vi "Periodic Tasks.vi"(8 "error in":errorcluster) -> ()   [LabVIEW 2018]
doc: "This VI runs in parallel to other tasks. It can contain as many user-defined periodic loops as you need. These can carry out PID or other sorts of timed response."
uses:
  State Machines/Intake.ctl
  State Machines/Climber.ctl
  <vilib>/Rock Robotics/WPI/Solenoid/WPI_SolenoidValue.ctl
  <vilib>/Rock Robotics/WPI/ThirdParty/Sensors/navX/_TypeDefs/FRIC_navX_DeviceNumbersTypeDef.ctl
  <vilib>/Rock Robotics/WPI/ThirdParty/Phoenix-LabVIEW/Motor Controller/Controls/CTRE_Phoenix_MotorControl_ControlMode.ctl
  Robot Global Data.vi
  Support Code/Valkyrie1Buttons.vi
  <vilib>/Rock Robotics/WPI/Utilities/WPI_GetSetVariantRefNum.vi
  <vilib>/Rock Robotics/WPI/Solenoid/WPI_SolenoidSetEnum.vi
  <vilib>/Rock Robotics/Network Tables/NT Write Number.vi
  <vilib>/Rock Robotics/Network Tables/NT Write Boolean.vi
panel:
  in  "Value":T1
  out "s? t:f":T1=enum."Forward"
  in  "Score Hatch Angle 2":dbl=12.0
  out "Climber State":T2=enum."cabou"
  in  "Retract back Speed":dbl=-0.4 format="%#_13g"
  in  "Retract Distance":dbl=1400.0 format="%#_13g"
  in  "Retract Speed":dbl=-0.1
  in  "Break speed":dbl=0.2 format="%#_13g"
  in  "Front Limit":dbl=1450.0 format="%#_13g"
  in  "Front Speed":dbl=1.0
  in  "Back Speed":dbl=0.9
  out "Encoder":i32=1460
  in  "Score Angle 2nd":dbl=1.0
  in  "Slow Mode":dbl=0.4
  in  "Cargo Deploy angle 2nd Floor":dbl=1.0
  in  "Cargo 2nd Floor Rocket":dbl=9.5
  in  "Cargo ship height":dbl=9.0
  in  "Cargo 1st Floor Rocket":dbl=5.0 format="%#_13g"
  out "elavador  pos":dbl=-0.00055775
  in  "Height  Hatch 2nd":dbl=9.0
  out "Intake pos":dbl=9.5952787399292
  in  "Turn on point multiplier":dbl=0.6 format="%#_13g"
  in  "Sensitivty":dbl=1.1 format="%#_13g"
  in  "Height Cargo Station":dbl=2.0
  in  "Height Cargo HP":dbl=9.0
  in  "Floor Angle Cargo":dbl=19.0
  in  "Gains":T3={"proportional gain (Kc)"=0.5, "integral time (Ti, min)"=0.1, "derivative time (Td, min)"=0.0} {"derivative time (Td, min)" format="%.3f"; "integral time (Ti, min)" format="%.3f"; "proportional gain (Kc)" format="%.3f"}
  in  "Range":cluster{"output high":dbl, "output low":dbl}={"output high"=1.0, "output low"=-0.4} {"output low" format="%.2f"; "output high" format="%.2f"}
  in  "Disable Range":dbl
  in  "Integral Range":dbl=1.0
  in  "CargoTime":dbl=10.0
  in  "Default height":dbl=3.0 format="%#_13g"
  in  "Cargo Deploy Angle":dbl=10.0
  in  "Tempo de coleta":dbl=7.0 format="%#_13g"
  in  "Sobe":dbl=1.0
  out "Estado Intake":T4
  in  "Desce":dbl=0.3
  in  "Score Hatch Angle":dbl=4.0 format="%#_13g"
  in  "Floor Angle":dbl=20.0
  in  "Hatch intake Speed Floor":dbl=-1.0
  in  "Holding Angle":dbl=4.0
  in  "Hatch intake Speed":dbl=-1.0
  in  "HP Angle 2":dbl=11.0 format="%#_13g"
  in  "HP Angle":dbl=10.0 format="%#_13g"
  in  "Intake Arm PID Constants":T5={"P Gain"=0.15, "I Gain"=1e-05, "D Gain"=5.0, "F Gain"=0.0, "I Zone"=10.0, "Min Output"=-0.2999999999999998, "Max Output"=0.3} {"Max Output" min=-1.0 max=1.0 step=0.01; "Min Output" min=-1.0 max=1.0 step=0.01; "I Zone" step=0.01; "F Gain" step=0.01; "D Gain" step=0.01; "I Gain" step=0.01; "P Gain" min=0.0 step=0.01}
  # "Angles"
  # "Intake Control"
  # "Elevator Control"
  # "Climber"
  # "Drivetrain"
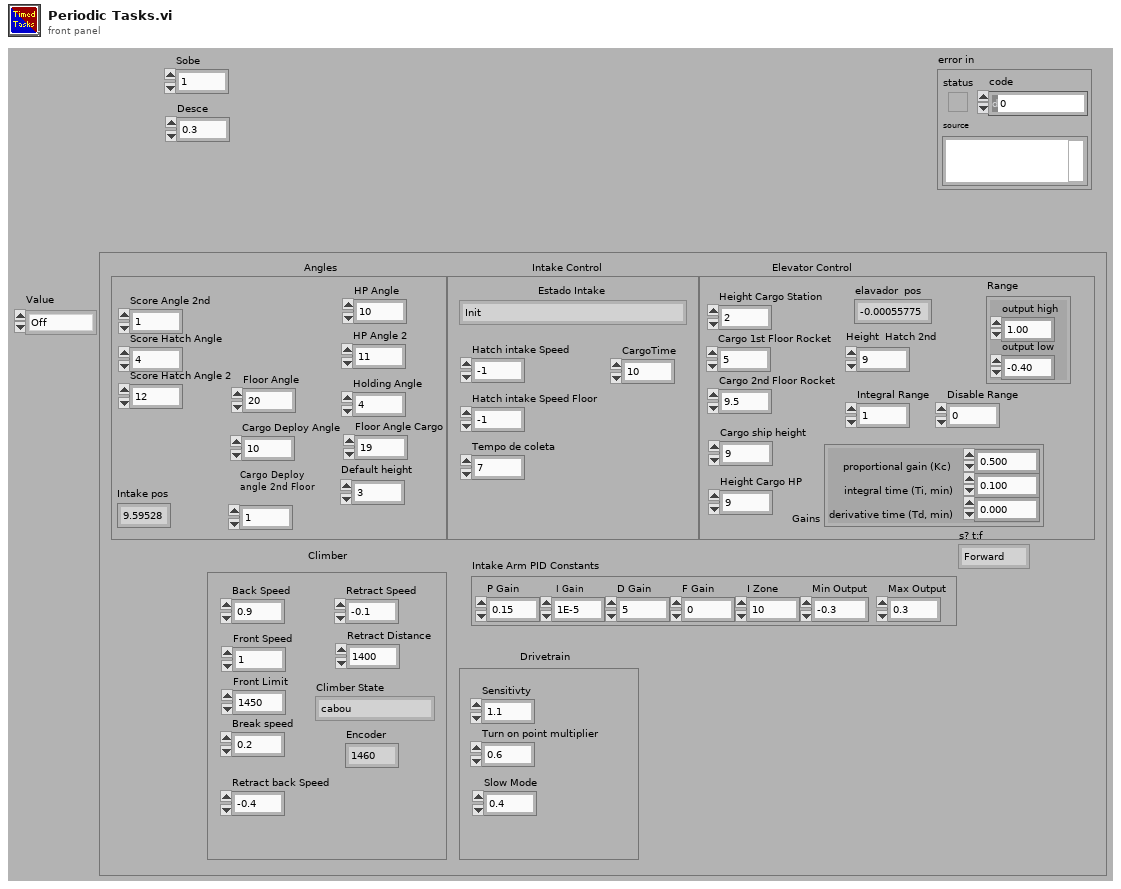
[diagram p1: front panel]
types:
  T1 = typedef "WPI_SolenoidValue.ctl" = enum16{"Off", "On", "Forward", "Reverse"}
  T2 = typedef "Climber.ctl" = enum16{"Engaging Climb", "Wait for Start", "ELEVATE!", "Hold position", "Forward", "Retract varetas", "Charge", "Sobe so um poquinho", "cabou"}
  T3 = cluster{"proportional gain (Kc)":dbl, "integral time (Ti, min)":dbl, "derivative time (Td, min)":dbl}
  T4 = typedef "Intake.ctl" = enum16{"Init", "Preparar Coletar HP", "Coletar Cargo", "Segurando Cargo", "Preparar Score Cargo", "Score Cargo", "Coletar HP", "Coletar Hatch Chão", "Segurando Hatch", "Preparar Score Hatch", "Score Hatch", "Wait"}
  T5 = cluster{"P Gain":dbl, "I Gain":dbl, "D Gain":dbl, "F Gain":dbl, "I Zone":dbl, "Min Output":dbl, "Max Output":dbl}
  T6 = typedef "FRIC_navX_DeviceNumbersTypeDef.ctl" = enum16{"Dev0", "Dev1", "Dev2", "Dev3"}
  T7 = typedef "WPI_MotorControlDeviceRef.ctl" = cluster{"DeviceStatus":errorcluster, "Type":T8, "PWM":cluster{"PWM Channel":T9, "DeadBand":T10}, "CAN":cluster{"Device Number":u8, "SetOutput VI Ref":variant, "GetOutput VI Ref":variant, "Enable VI Ref":variant, "Disable VI Ref":variant, "Data":variant}, "Invert":bool, "DIO PWM":cluster{"PWM \"Enable\" Channel":T9, "DIOChannel":T11, "PWM Rate":dbl}}
  T8 = typedef "WPI_MotorControlType.ctl" = enum16{"PWM", "CAN", "DIO PWM"}
  T9 = typedef "FPGA_DIOPWMChannel.ctl" = enum8{"PWM 0", "PWM 1", "PWM 2", "PWM 3", "PWM 4", "PWM 5", "PWM 6", "PWM 7", "PWM 8", "PWM 9", "PWM MXP 0", "PWM MXP 1", "PWM MXP 2", "PWM MXP 3", "PWM MXP 4", "PWM MXP 5", "PWM MXP 6", "PWM MXP 7", "PWM MXP 8", "PWM MXP 9", "Invalid"}
  T10 = typedef "WPI_PWMDeadband.ctl" = cluster{"Name":string, "maxPositivePwm":i32, "minPositivePwm":i32, "centerPwm":i32, "maxNegativePwm":i32, "minNegativePwm":i32, "angularRange":u16}
  T11 = typedef "FPGA_DIOChannel.ctl" = enum8{"DIO 0", "DIO 1", "DIO 2", "DIO 3", "DIO 4", "DIO 5", "DIO 6", "DIO 7", "DIO 8", "DIO 9", "DIO MXP 0", "DIO MXP 1", "DIO MXP 2", "DIO MXP 3", "DIO MXP 4", "DIO MXP 5", "DIO MXP 6", "DIO MXP 7", "DIO MXP 8", "DIO MXP 9", "DIO MXP 10", "DIO MXP 11", "DIO MXP 12", "DIO MXP 13", "DIO MXP 14", "DIO MXP 15", "SPI Port CS1", "SPI Port CS2", "SPI Port CS3", "SPI Port MISO", "SPI Port MOSI", "Invalid"}
  T12 = typedef "Button Cluster.ctl" = cluster{"Buttons[0]":bool, "Buttons[1]":bool, "Buttons[2]":bool, "Buttons[3]":bool, "Buttons[4]":bool, "Buttons[5]":bool, "Buttons[6]":bool, "Buttons[7]":bool, "Buttons[8]":bool, "Buttons[9]":bool}
  T13 = typedef "WPI_SwitchDevRef.ctl" = cluster{"DevStatus":errorcluster, "DIO Channel":T11, "CntIndex":T14, "Normally Closed":bool}
  T14 = typedef "FPGA_CounterCtrSystemIndex.ctl" = enum8{"Ctr 0", "Ctr 1", "Ctr 2", "Ctr 3", "Ctr 4", "Ctr 5", "Ctr 6", "Ctr 7", "Invalid"}
  T15 = typedef "WPI_SolenoidDevRef.ctl" = cluster{"DevStatus":errorcluster, "Pneumatics Control Module":u8, "Forward Solenoid Channel":T16, "Reverse Solenoid Channel":T16}
  T16 = typedef "WPI_SolenoidChannel.ctl" = enum8{"Solenoid 0", "Solenoid 1", "Solenoid 2", "Solenoid 3", "Solenoid 4", "Solenoid 5", "Solenoid 6", "Solenoid 7", "Invalid"}
  T17 = typedef "WPI_EncoderDevRef.ctl" = cluster{"DevStatus":errorcluster, "EncoderIndex":T18, "CounterIndex":T14, "DistancePerCount":dbl, "Decoding Type":T19}
  T18 = typedef "FPGA_EncoderIdx.ctl" = enum8{"Enc 0", "Enc 1", "Enc 2", "Enc 3", "Enc 4", "Enc 5", "Enc 6", "Enc 7", "Invalid"}
  T19 = typedef "WPI_EncoderType.ctl" = enum16{"1x", "2x", "4x"}
  T20 = typedef "CTRE_Phoenix_MotorControl_ControlMode.ctl" = u16
  T21 = typedef "WPI_CounterDevRef.ctl" = cluster{"DevStatus":errorcluster, "CntIndex":T14}
  T22 = typedef "WPI_RobotDriveDevRef.ctl" = cluster{"DevStatus":errorcluster, "Motors[]":T7[], "Square Inputs":bool, "Max Output":dbl}
  T23 = typedef "Axes Cluster.ctl" = cluster{"Axes[0]":dbl, "Axes[1]":dbl, "Axes[2]":dbl, "Axes[3]":dbl, "Axes[4]":dbl, "Axes[5]":dbl, "Axes[6]":dbl, "Axes[7]":dbl, "Axes[8]":dbl}
  T24 = typedef "D-Pad.ctl" = cluster{"Top":bool, "Bottom":bool, "None":bool, "Right":bool, "Left":bool}
  T25 = typedef "WPI_CompressorDevRef.ctl" = cluster{"DevStatus":errorcluster, "Pneumatics Control Module":u8}
  T26 = typedef "WPI_JoystickDevRef.ctl" = cluster{"Device":T27}
  T27 = typedef "WPI_JoystickDeviceEnum.ctl" = enum16{"USB 0", "USB 1", "USB 2", "USB 3", "USB 4", "USB 5"}
  T28 = cluster{"Rollover":dbl, "Yaw":dbl, "Cont Yaw":dbl}
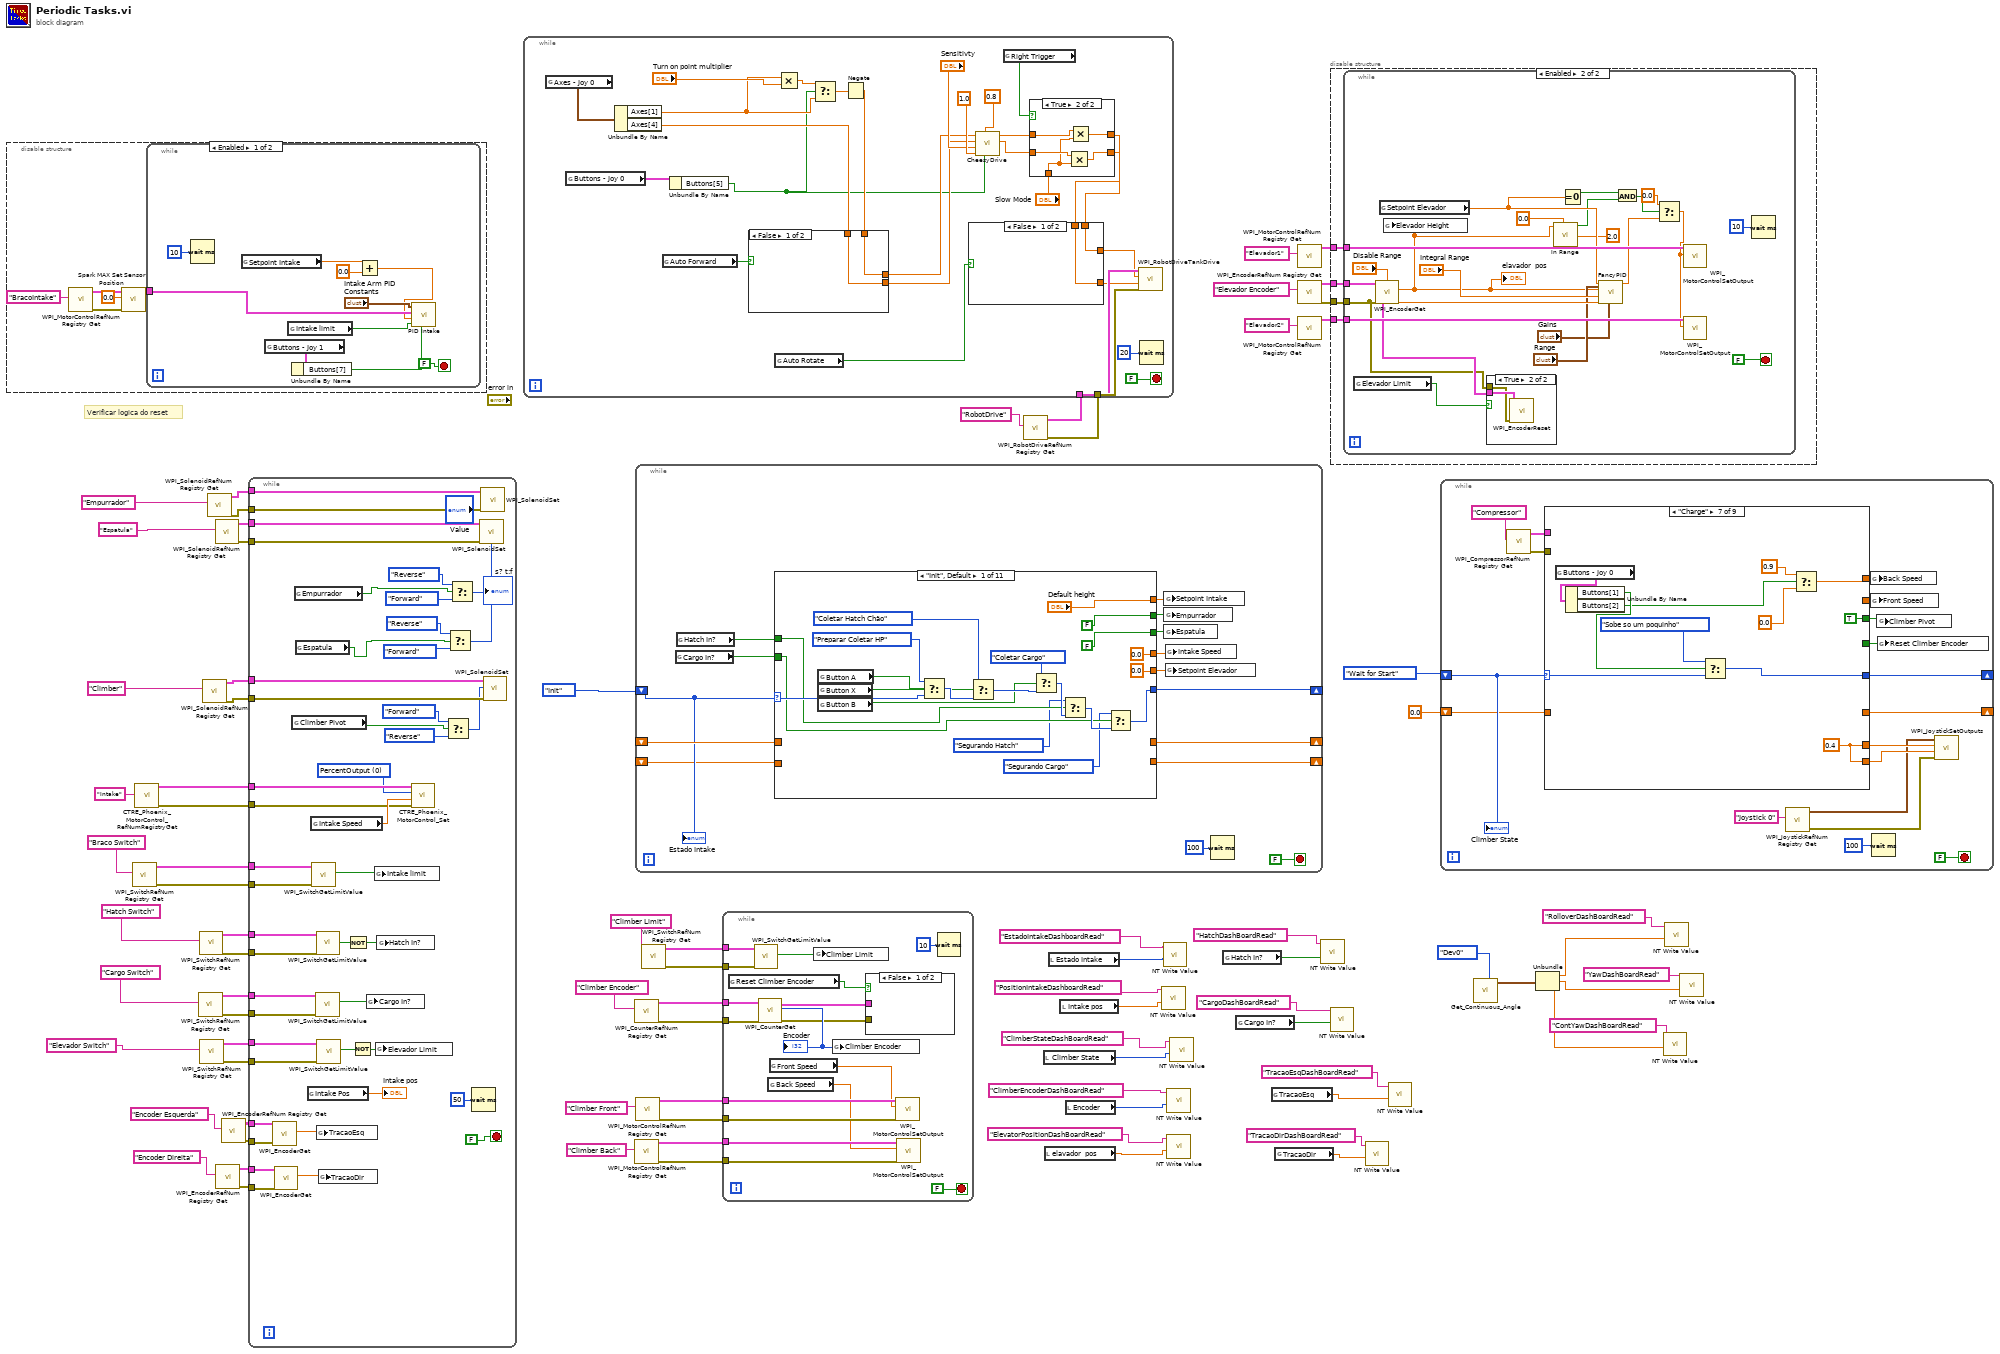
[diagram p0: block diagram]
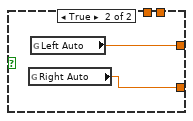
[diagram p2: hidden frame]
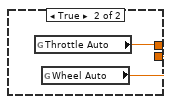
[diagram p3: hidden frame]
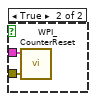
[diagram p5: hidden frame]
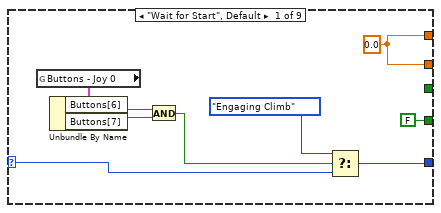
[diagram p6: hidden frame]
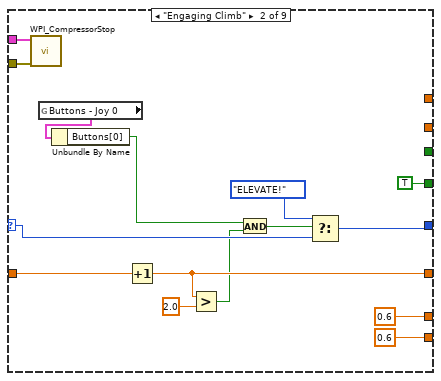
[diagram p7: hidden frame]
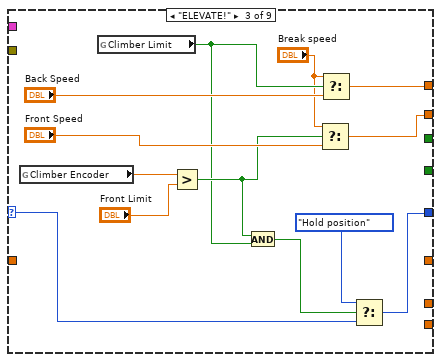
[diagram p8: hidden frame]
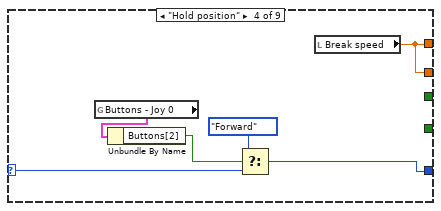
[diagram p9: hidden frame]
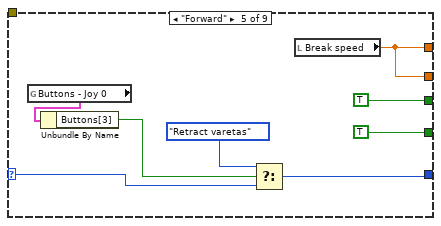
[diagram p10: hidden frame]
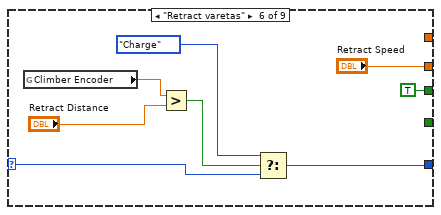
[diagram p11: hidden frame]
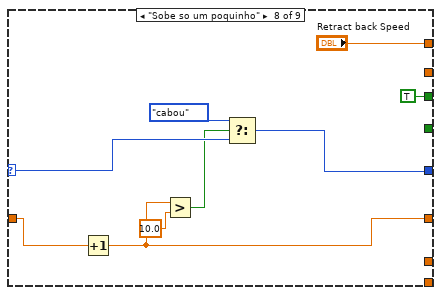
[diagram p12: hidden frame]
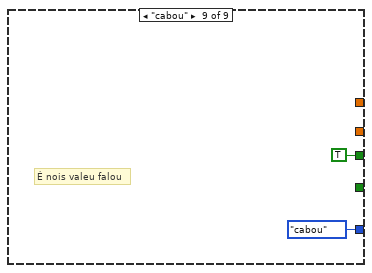
[diagram p13: hidden frame]
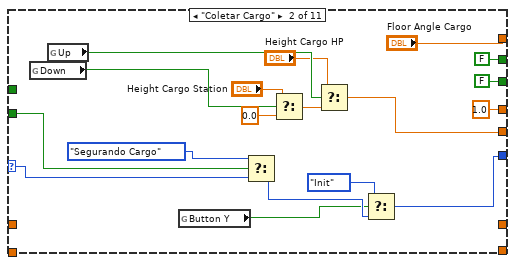
[diagram p14: hidden frame]
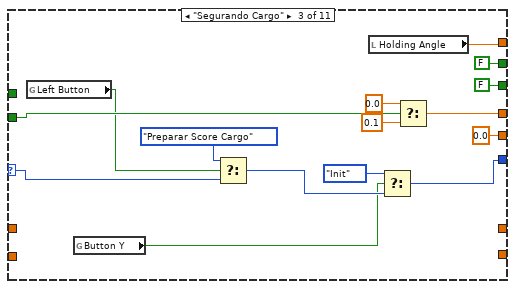
[diagram p15: hidden frame]
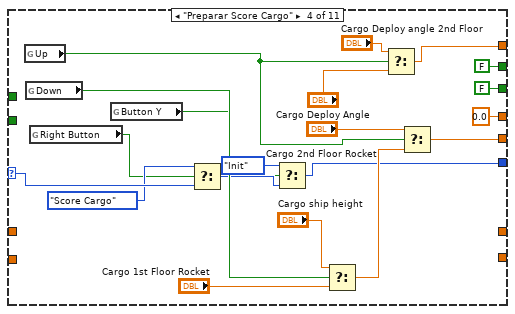
[diagram p16: hidden frame]
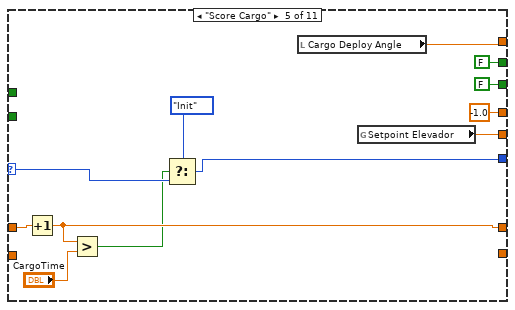
[diagram p17: hidden frame]
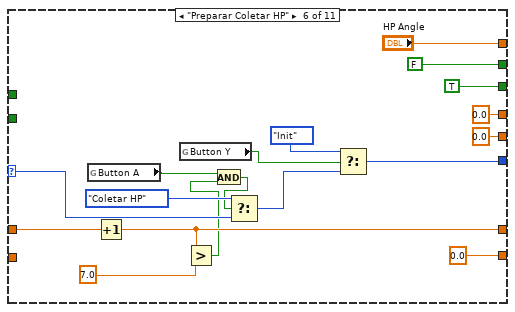
[diagram p18: hidden frame]
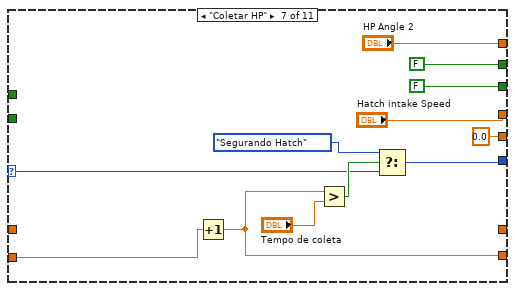
[diagram p19: hidden frame]
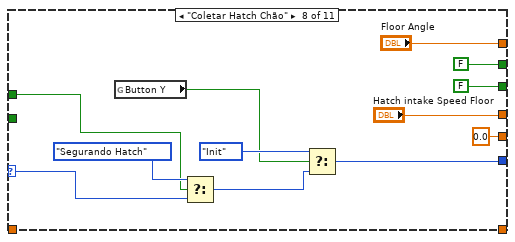
[diagram p20: hidden frame]
diagram:
  # "Verificar logica do reset"
  n1 = disable-structure shown="Enabled" {
    frame Enabled {
      n2 = call <vilib>:"WPI_MotorControlRefNum Registry Get.vi"("refnum name"="BracoIntake") -> ("error out"=w83:errorcluster, "MotorControlDevRef"=w84:T7)  [unwired: 9 in]
      n3 = call <vilib>:"Spark MAX Set Sensor Position.vi"("error in"=w83, "Position"=0.0, "MotorControlDeviceRef"=w84) -> ("MotorControlDeviceRef"=w85:T7)  [unwired: 7 in, 1 out]
      n4 = while {
        tunnel: w85 -> [w94]
        stop <- FALSE stop-if-true
        n5 = Wait (ms)(milliseconds to wait=u32 10) -> ()  [unwired: 1 out]
        n6 = global read "Robot Global Data.vi" "Setpoint Intake"() -> (w89:dbl)
        n7 = global read "Robot Global Data.vi" "Buttons - Joy 1"() -> (w92:T12)
        n8 = global read "Robot Global Data.vi" "Intake limit"() -> (w90:bool)
        n9 = Unbundle By Name(w92) -> ("Buttons[7]"=w91:bool)
        n10 = Add(x=w89, y=0.0) -> (x+y=w88:dbl)
        n11 = call "PID Intake.vi"("Encoder Overide"=w91, "Limit"=w90, "Setpoint Intake"=w88, "MotorControlDevRef"=w94, "PID Constants"="Intake Arm PID Constants") -> ()  [unwired: 7 in]
      }
    }
    frame Disabled {
    }
  }
  n12 = call <vilib>:"WPI_SwitchRefNum Registry Get.vi"("refnum name"="Braco Switch") -> ("error out"=w77:errorcluster, "SwitchDevRef"=w78:T13)  [unwired: 9 in]
  n13 = call <vilib>:"CTRE_Phoenix_MotorControl_RefNumRegistryGet.vi"("refnum name"="Intake") -> ("error out"=w73:errorcluster, "PhoenixMotorControlDevRef"=w74:T7)  [unwired: 9 in]
  n14 = call <vilib>:"WPI_SwitchRefNum Registry Get.vi"("refnum name"="Cargo Switch") -> ("error out"=w64:errorcluster, "SwitchDevRef"=w65:T13)  [unwired: 9 in]
  n15 = call <vilib>:"WPI_SwitchRefNum Registry Get.vi"("refnum name"="Hatch Switch") -> ("error out"=w72:errorcluster, "SwitchDevRef"=w71:T13)  [unwired: 9 in]
  n16 = call <vilib>:"WPI_SwitchRefNum Registry Get.vi"("refnum name"="Elevador Switch") -> ("error out"=w52:errorcluster, "SwitchDevRef"=w51:T13)  [unwired: 9 in]
  n17 = call <vilib>:"WPI_SolenoidRefNum Registry Get.vi"("refnum name"="Climber") -> ("error out"=w68:errorcluster, "SolenoidDevRef"=w67:T15)  [unwired: 9 in]
  n18 = call <vilib>:"WPI_SolenoidRefNum Registry Get.vi"("refnum name"="Empurrador") -> ("error out"=w62:errorcluster, "SolenoidDevRef"=w61:T15)  [unwired: 9 in]
  n19 = call <vilib>:"WPI_SolenoidRefNum Registry Get.vi"("refnum name"="Espatula") -> ("error out"=w79:errorcluster, "SolenoidDevRef"=w80:T15)  [unwired: 9 in]
  n20 = call <vilib>:"WPI_EncoderRefNum Registry Get.vi"("refnum name"="Encoder Direita") -> ("error out"=w1:errorcluster, "EncoderDevRef"=w2:T17)  [unwired: 9 in]
  n21 = call <vilib>:"WPI_EncoderRefNum Registry Get.vi"("refnum name"="Encoder Esquerda") -> ("error out"=w4:errorcluster, "EncoderDevRef"=w5:T17)  [unwired: 9 in]
  n22 = while {
    tunnel: w61 -> [w142]
    tunnel: w62 -> [w141]
    tunnel: w80 -> [w140]
    tunnel: w79 -> [w139]
    tunnel: w67 -> [w138]
    tunnel: w68 -> [w137]
    tunnel: w74 -> [w125]
    tunnel: w78 -> [w122]
    tunnel: w77 -> [w121]
    tunnel: w73 -> [w120]
    tunnel: w71 -> [w118]
    tunnel: w72 -> [w119]
    tunnel: w65 -> [w114]
    tunnel: w64 -> [w113]
    tunnel: w51 -> [w108]
    tunnel: w52 -> [w109]
    tunnel: w4 -> [w102]
    tunnel: w2 -> [w100]
    tunnel: w1 -> [w99]
    tunnel: w5 -> [w97]
    stop <- FALSE stop-if-true
    w124 = T20 0 items=["PercentOutput"=0, "Position"=1, "Velocity"=2, "Current"=3, "Follower"=5, "MotionProfile"=6, "MotionMagic"=7, "MotionProfileArc"=10, "Disabled"=15] ("Control Mode")
    n23 = call <vilib>:"WPI_EncoderGet.vi"("error in (no error)"=w102, "EncoderDevRef"=w97) -> ("Distance"=w101:dbl)  [unwired: 4 in, 5 out]
    n24 = call <vilib>:"WPI_EncoderGet.vi"("error in (no error)"=w99, "EncoderDevRef"=w100) -> ("Distance"=w98:dbl)  [unwired: 4 in, 5 out]
    n25 = global read "Robot Global Data.vi" "Climber Pivot"() -> (w126:bool)
    n26 = global read "Robot Global Data.vi" "Empurrador"() -> (w115:bool)
    n27 = global read "Robot Global Data.vi" "Espatula"() -> (w116:bool)
    n28 = global read "Robot Global Data.vi" "Intake Pos"() -> (→"Intake pos":dbl)
    n29 = global read "Robot Global Data.vi" "Intake Speed"() -> (w123:dbl)
    n30 = call <vilib>:"WPI_SwitchGetLimitValue.vi"("error in (no error)"=w121, "SwitchDevRef"=w122) -> ("Switch Pressed"=w106:bool)  [unwired: 7 in, 2 out]
    n31 = call <vilib>:"WPI_SwitchGetLimitValue.vi"("error in (no error)"=w113, "SwitchDevRef"=w114) -> ("Switch Pressed"=w105:bool)  [unwired: 7 in, 2 out]
    n32 = call <vilib>:"WPI_SwitchGetLimitValue.vi"("error in (no error)"=w119, "SwitchDevRef"=w118) -> ("Switch Pressed"=w117:bool)  [unwired: 7 in, 2 out]
    n33 = global write "Robot Global Data.vi" "TracaoEsq"(w101) -> ()
    n34 = call <vilib>:"WPI_SwitchGetLimitValue.vi"("error in (no error)"=w109, "SwitchDevRef"=w108) -> ("Switch Pressed"=w110:bool)  [unwired: 7 in, 2 out]
    n35 = global write "Robot Global Data.vi" "TracaoDir"(w98) -> ()
    n36 = Not(x=w117) -> (.not. x?=w112:bool)
    n37 = Not(x=w110) -> (.not. x?=w107:bool)
    n38 = global write "Robot Global Data.vi" "Cargo In?"(w105) -> ()
    n39 = global write "Robot Global Data.vi" "Intake limit"(w106) -> ()
    n40 = global write "Robot Global Data.vi" "Elevador Limit"(w107) -> ()
    n41 = global write "Robot Global Data.vi" "Hatch In?"(w112) -> ()
    n42 = call <vilib>:"CTRE_Phoenix_MotorControl_Set.vi"("error in (no error)"=w120, "Output"=w123, "Control Mode"=w124, "PhoenixMotorControlDevRef"=w125) -> ()  [unwired: 6 in, 2 out]
    n43 = Select(t=WPI_SolenoidValue."Forward" ("Value"), s=w126, f=WPI_SolenoidValue."Reverse") -> (s? t:f=w132:T1)
    n44 = Select(t=WPI_SolenoidValue."Reverse" ("Value"), s=w116, f=WPI_SolenoidValue."Forward") -> (s? t:f=w129:T1)
    n45 = Select(t=WPI_SolenoidValue."Reverse" ("Value"), s=w115, f=WPI_SolenoidValue."Forward") -> (s? t:f=→"s? t:f":T1)
    n46 = Wait (ms)(milliseconds to wait=u32 50) -> ()  [unwired: 1 out]
    n47 = call-poly <vilib>:"WPI_SolenoidSet.vi"("error in (no error)"=w139, "Value"=w129, "SolenoidDevRef"=w140) -> ()  [unwired: 7 in, 2 out]
    n48 = call-poly <vilib>:"WPI_SolenoidSet.vi"("error in (no error)"=w141, "Value"="Value", "SolenoidDevRef"=w142) -> ()  [unwired: 7 in, 2 out]
    n49 = call-poly <vilib>:"WPI_SolenoidSet.vi"("error in (no error)"=w137, "Value"=w132, "SolenoidDevRef"=w138) -> ()  [unwired: 7 in, 2 out]
  }
  n50 = call <vilib>:"WPI_CounterRefNum Registry Get.vi"("refnum name"="Climber Encoder") -> ("error out"=w43:errorcluster, "CounterDevRef"=w44:T21)  [unwired: 9 in]
  n51 = call <vilib>:"WPI_MotorControlRefNum Registry Get.vi"("refnum name"="Climber Back") -> ("error out"=w37:errorcluster, "MotorControlDevRef"=w39:T7)  [unwired: 9 in]
  n52 = while {
    shift-right: [w156] -> _
    shift-left: Intake."Init" -> [w152]
    shift-right: [w153] -> _
    shift-left: _ -> [w154]
    shift-right: [w150] -> _
    shift-left: _ -> [w149]
    stop <- FALSE stop-if-true
    n53 = global read "Robot Global Data.vi" "Cargo In?"() -> (w143:bool)
    n54 = global read "Robot Global Data.vi" "Hatch In?"() -> (w151:bool)
    n55 = case shown="\"Init\", Default" w152 {
      selector: w152 -> [w175 w186 w211 w228 w234 w261 w269 w277 w289 w312 w320]
      tunnel: ["Default height" "Floor Angle Cargo" w204 w216 w243 "HP Angle" "HP Angle 2" "Floor Angle" "Holding Angle" w300 "Score Hatch Angle 2"] -> w148
      tunnel: [FALSE FALSE FALSE FALSE FALSE FALSE FALSE FALSE FALSE FALSE TRUE] -> w147
      tunnel: [FALSE FALSE FALSE FALSE FALSE TRUE FALSE FALSE FALSE FALSE TRUE] -> w146
      tunnel: [w164 w187 w200 w214 w239 w259 w272 w280 w293 w309 w319] -> w156
      tunnel: w154 -> [_ _ _ _ w238 w251 _ _ _ _ _]
      tunnel: [_ _ _ _ w237 w256 _ _ _ _ _] -> w153
      tunnel: [0.0 ("Hatch intake Speed Floor") 1.0 ("Hatch intake Speed Floor") w210 0.0 ("Hatch intake Speed Floor") -1.0 ("Hatch intake Speed Floor") 0.0 ("Hatch intake Speed Floor") "Hatch intake Speed" "Hatch intake Speed Floor" -0.1 ("Hatch intake Speed Floor") 0.0 ("Hatch intake Speed Floor") 0.0 ("Hatch intake Speed Floor")] -> w145
      tunnel: w151 -> [w161 _ _ _ _ _ _ w276 _ _ _]
      tunnel: [_ _ _ _ _ 0.0 ("y") w263 _ _ _ _] -> w150
      tunnel: w149 -> [_ _ _ _ _ _ w264 _ _ _ _]
      tunnel: [0.0 ("ElevadorRocket") w196 0.0 ("ElevadorRocket") w221 w235 0.0 ("ElevadorRocket") 0.0 ("ElevadorRocket") 0.0 ("ElevadorRocket") 0.0 ("ElevadorRocket") w303 w316] -> w144
      tunnel: w143 -> [w160 w190 w209 _ _ _ _ _ _ _ _]
      frame "Init", Default {
        n56 = global read "Valkyrie1Buttons.vi" "Button A"() -> (w165:bool)
        n57 = global read "Valkyrie1Buttons.vi" "Button X"() -> (w167:bool)
        n58 = global read "Valkyrie1Buttons.vi" "Button B"() -> (w166:bool)
        n59 = Select(t=Intake."Preparar Coletar HP", s=w165, f=w175) -> (s? t:f=w174:T4)
        n60 = Select(t=Intake."Coletar Hatch Chão", s=w167, f=w174) -> (s? t:f=w169:T4)
        n61 = Select(t=Intake."Coletar Cargo", s=w166, f=w169) -> (s? t:f=w163:T4)
        n62 = Select(t=Intake."Segurando Hatch", s=w161, f=w163) -> (s? t:f=w162:T4)
        n63 = Select(t=Intake."Segurando Cargo", s=w160, f=w162) -> (s? t:f=w164:T4)
      }
      frame "Coletar Cargo" {
        n64 = global read "Valkyrie1Buttons.vi" "Down"() -> (w184:bool)
        n65 = global read "Valkyrie1Buttons.vi" "Up"() -> (w185:bool)
        n66 = global read "Valkyrie1Buttons.vi" "Button Y"() -> (w183:bool)
        n67 = Select(t=Intake."Segurando Cargo", s=w190, f=w186) -> (s? t:f=w188:T4)
        n68 = Select(t="Height Cargo Station", s=w184, f=0.0) -> (s? t:f=w195:dbl)
        n69 = Select(t="Height Cargo HP", s=w185, f=w195) -> (s? t:f=w196:dbl)
        n70 = Select(t=Intake."Init", s=w183, f=w188) -> (s? t:f=w187:T4)
      }
      frame "Segurando Cargo" {
        n71 = global read "Valkyrie1Buttons.vi" "Left Button"() -> (w202:bool)
        n72 = global read "Valkyrie1Buttons.vi" "Button Y"() -> (w198:bool)
        n73 = Select(t=Intake."Preparar Score Cargo", s=w202, f=w211) -> (s? t:f=w199:T4)
        n74 = local read "Holding Angle"() -> (w204:dbl)
        n75 = Select(t=Intake."Init", s=w198, f=w199) -> (s? t:f=w200:T4)
        n76 = Select(t=0.0, s=w209, f=0.1) -> (s? t:f=w210:dbl)
      }
      frame "Preparar Score Cargo" {
        n77 = global read "Valkyrie1Buttons.vi" "Up"() -> (w217:bool)
        n78 = global read "Valkyrie1Buttons.vi" "Down"() -> (w220:bool)
        n79 = global read "Valkyrie1Buttons.vi" "Right Button"() -> (w226:bool)
        n80 = global read "Valkyrie1Buttons.vi" "Button Y"() -> (w213:bool)
        n81 = Select(t=Intake."Score Cargo", s=w226, f=w228) -> (s? t:f=w215:T4)
        n82 = Select(t=Intake."Init", s=w213, f=w215) -> (s? t:f=w214:T4)
        n83 = Select(t="Cargo ship height", s=w220, f="Cargo 1st Floor Rocket") -> (s? t:f=w224:dbl)
        n84 = Select(t="Cargo Deploy angle 2nd Floor", s=w217, f="Cargo Deploy Angle") -> (s? t:f=w216:dbl)
        n85 = Select(t="Cargo 2nd Floor Rocket", s=w217, f=w224) -> (s? t:f=w221:dbl)
      }
      frame "Score Cargo" {
        n86 = Increment(x=w238) -> (x+1=w237:dbl)
        n87 = Greater?(x=w237, y="CargoTime") -> (0:w232:bool)
        n88 = Select(t=Intake."Init", s=w232, f=w234) -> (s? t:f=w239:T4)
        n89 = local read "Cargo Deploy Angle"() -> (w243:dbl)
        n90 = global read "Robot Global Data.vi" "Setpoint Elevador"() -> (w235:dbl)
      }
      frame "Preparar Coletar HP" {
        n91 = global read "Valkyrie1Buttons.vi" "Button A"() -> (w245:bool)
        n92 = Increment(x=w251) -> (x+1=w256:dbl)
        n93 = global read "Valkyrie1Buttons.vi" "Button Y"() -> (w244:bool)
        n94 = Greater?(x=w256, y=7.0) -> (0:w248:bool)
        n95 = And(x=w245, y=w248) -> (x .and. y?=w247:bool)
        n96 = Select(t=Intake."Coletar HP", s=w247, f=w261) -> (s? t:f=w260:T4)
        n97 = Select(t=Intake."Init", s=w244, f=w260) -> (s? t:f=w259:T4)
      }
      frame "Coletar HP" {
        n98 = Increment(x=w264) -> (x+1=w263:dbl)
        n99 = Greater?(x=w263, y="Tempo de coleta") -> (0:w270:bool)
        n100 = Select(t=Intake."Segurando Hatch", s=w270, f=w269) -> (s? t:f=w272:T4)
      }
      frame "Coletar Hatch Chão" {
        n101 = global read "Valkyrie1Buttons.vi" "Button Y"() -> (w274:bool)
        n102 = Select(t=Intake."Segurando Hatch", s=w276, f=w277) -> (s? t:f=w279:T4)
        n103 = Select(t=Intake."Init", s=w274, f=w279) -> (s? t:f=w280:T4)
      }
      frame "Segurando Hatch" {
        n104 = global read "Valkyrie1Buttons.vi" "Left Button"() -> (w286:bool)
        n105 = global read "Valkyrie1Buttons.vi" "Button Y"() -> (w287:bool)
        n106 = Select(t=Intake."Preparar Score Hatch", s=w286, f=w289) -> (s? t:f=w291:T4)
        n107 = Select(t=Intake."Init", s=w287, f=w291) -> (s? t:f=w293:T4)
      }
      frame "Preparar Score Hatch" {
        n108 = global read "Valkyrie1Buttons.vi" "Up"() -> (w299:bool)
        n109 = global read "Valkyrie1Buttons.vi" "Right Button"() -> (w306:bool)
        n110 = global read "Valkyrie1Buttons.vi" "Button Y"() -> (w305:bool)
        n111 = Select(t=Intake."Score Hatch", s=w306, f=w312) -> (s? t:f=w310:T4)
        n112 = Select(t=Intake."Init", s=w305, f=w310) -> (s? t:f=w309:T4)
        n113 = Select(t="Height  Hatch 2nd", s=w299, f=0.0) -> (s? t:f=w303:dbl)
        n114 = Select(t="Score Angle 2nd", s=w299, f="Score Hatch Angle") -> (s? t:f=w300:dbl)
      }
      frame "Score Hatch" {
        n115 = global read "Valkyrie1Buttons.vi" "Button Y"() -> (w317:bool)
        n116 = Select(t=Intake."Init", s=w317, f=w320) -> (s? t:f=w319:T4)
        n117 = global read "Robot Global Data.vi" "Setpoint Elevador"() -> (w316:dbl)
      }
    }
    n118 = global write "Robot Global Data.vi" "Setpoint Intake"(w148) -> ()
    n119 = global write "Robot Global Data.vi" "Empurrador"(w147) -> ()
    n120 = global write "Robot Global Data.vi" "Espatula"(w146) -> ()
    n121 = global write "Robot Global Data.vi" "Intake Speed"(w145) -> ()
    n122 = global write "Robot Global Data.vi" "Setpoint Elevador"(w144) -> ()
    n123 = Wait (ms)(milliseconds to wait=u32 100) -> ()  [unwired: 1 out]
    "Estado Intake" <- w152
  }
  n124 = call <vilib>:"WPI_MotorControlRefNum Registry Get.vi"("refnum name"="Climber Front") -> ("error out"=w38:errorcluster, "MotorControlDevRef"=w40:T7)  [unwired: 9 in]
  n125 = call <vilib>:"WPI_SwitchRefNum Registry Get.vi"("refnum name"="Climber Limit") -> ("error out"=w47:errorcluster, "SwitchDevRef"=w48:T13)  [unwired: 9 in]
  n126 = while {
    tunnel: w48 -> [w338]
    tunnel: w47 -> [w337]
    tunnel: w44 -> [w336]
    tunnel: w43 -> [w335]
    tunnel: w40 -> [w333]
    tunnel: w39 -> [w332]
    tunnel: w38 -> [w331]
    tunnel: w37 -> [w330]
    stop <- FALSE stop-if-true
    n127 = global read "Robot Global Data.vi" "Reset Climber Encoder"() -> (w325:bool)
    n128 = call <vilib>:"WPI_SwitchGetLimitValue.vi"("error in (no error)"=w337, "SwitchDevRef"=w338) -> ("Switch Pressed"=w326:bool)  [unwired: 7 in, 2 out]
    n129 = call <vilib>:"WPI_CounterGet.vi"("error in (no error)"=w335, "CounterDevRef in"=w336) -> ("error out"=w327:errorcluster, "Value"=w334:i32, "CounterDevRef out"=w328:T21)  [unwired: 4 in, 3 out]
    "Encoder" <- w334
    n130 = global read "Robot Global Data.vi" "Back Speed"() -> (w329:dbl)
    n131 = global read "Robot Global Data.vi" "Front Speed"() -> (w324:dbl)
    n132 = global write "Robot Global Data.vi" "Climber Limit"(w326) -> ()
    n133 = global write "Robot Global Data.vi" "Climber Encoder"(w334) -> ()
    n134 = case shown="False" w325 {
      tunnel: w328 -> [_ w342]
      tunnel: w327 -> [_ w341]
      frame False {
      }
      frame True {
        n135 = call <vilib>:"WPI_CounterReset.vi"("error in (no error)"=w341, "CounterDevRef in"=w342) -> ()  [unwired: 8 in, 2 out]
      }
    }
    n136 = call <vilib>:"WPI_MotorControlSetOutput.vi"("error in (no error)"=w331, "Output"=w324, "MotorControlDevRef"=w333) -> ()  [unwired: 6 in, 3 out]
    n137 = call <vilib>:"WPI_MotorControlSetOutput.vi"("error in (no error)"=w330, "Output"=w329, "MotorControlDevRef"=w332) -> ()  [unwired: 6 in, 3 out]
    n138 = Wait (ms)(milliseconds to wait=u32 10) -> ()  [unwired: 1 out]
  }
  n139 = call <vilib>:"WPI_RobotDriveRefNum Registry Get.vi"("refnum name"="RobotDrive") -> ("error out"=w35:errorcluster, "RobotDriveDevRef"=w34:T22)  [unwired: 9 in]
  n140 = while {
    tunnel: w35 -> [w367]
    tunnel: w34 -> [w366]
    stop <- FALSE stop-if-true
    n141 = global read "Robot Global Data.vi" "Axes - Joy 0"() -> (w369:T23)
    n142 = global read "Robot Global Data.vi" "Buttons - Joy 0"() -> (w344:T12)
    n143 = Unbundle By Name(w369) -> ("Axes[1]"=w359:dbl, "Axes[4]"=w351:dbl)
    n144 = global read "Robot Global Data.vi" "Auto Forward"() -> (w350:bool)
    n145 = Unbundle By Name(w344) -> ("Buttons[5]"=w343:bool)
    n146 = global read "Robot Global Data.vi" "Auto Rotate"() -> (w345:bool)
    n147 = Multiply(x=w359, y="Turn on point multiplier") -> (x*y=w362:dbl)
    n148 = Select(t=w362, s=w343, f=w359) -> (s? t:f=w360:dbl)
    n149 = Negate(x=w360) -> (-x=w353:dbl)
    n150 = case shown="False" w350 {
      tunnel: [w376 w378] -> w354
      tunnel: [w375 w377] -> w352
      tunnel: w353 -> [w376 _]
      tunnel: w351 -> [w375 _]
      frame False {
      }
      frame True {
        n151 = global read "Robot Global Data.vi" "Throttle Auto"() -> (w378:dbl)
        n152 = global read "Robot Global Data.vi" "Wheel Auto"() -> (w377:dbl)
      }
    }
    n153 = call "CheesyDrive.vi"("Quickturn"=w343, "WheelNonLinearity"=0.8, "negInertiaScalar"=1.0, "Sensitivty"="Sensitivty", "Wheel"=w352, "Throttle"=w354) -> ("Right PWM"=w356:dbl, "Left PWM"=w357:dbl)  [unwired: 4 in]
    n154 = global read "Valkyrie1Buttons.vi" "Right Trigger"() -> (w358:bool)
    n155 = case shown="True" w358 {
      tunnel: w357 -> [w380 w383]
      tunnel: [w380 w385] -> w347
      tunnel: w356 -> [w379 w382]
      tunnel: [w379 w384] -> w346
      tunnel: "Slow Mode" -> [_ w381]
      frame False {
      }
      frame True {
        n156 = Multiply(x=w382, y=w381) -> (x*y=w384:dbl)
        n157 = Multiply(x=w383, y=w381) -> (x*y=w385:dbl)
      }
    }
    n158 = case shown="False" w345 {
      tunnel: [w372 w374] -> w349
      tunnel: [w371 w373] -> w348
      tunnel: w347 -> [w372 _]
      tunnel: w346 -> [w371 _]
      frame False {
      }
      frame True {
        n159 = global read "Robot Global Data.vi" "Right Auto"() -> (w373:dbl)
        n160 = global read "Robot Global Data.vi" "Left Auto"() -> (w374:dbl)
      }
    }
    n161 = call <vilib>:"WPI_RobotDriveTankDrive.vi"("error in (no error)"=w367, "Right axis value"=w348, "Left axis value"=w349, "RobotDriveDevRef"=w366) -> ()  [unwired: 5 in, 3 out]
    n162 = Wait (ms)(milliseconds to wait=u32 20) -> ()  [unwired: 1 out]
  }
  n163 = local read "Climber State"() -> (w19:T2)
  n164 = local read "elavador  pos"() -> (w27:dbl)
  n165 = local read "Estado Intake"() -> (w23:T4)
  n166 = local read "Intake pos"() -> (w21:dbl)
  n167 = local read "Encoder"() -> (w25:i32)
  n168 = call-poly <vilib>:"NT Write Value.vi"("Numeric"=w21, "Name"="PositionIntakeDashboardRead") -> ()  [unwired: 9 in, 1 out]
  n169 = call-poly <vilib>:"NT Write Value.vi"("Numeric"=w23, "Name"="EstadoIntakeDashboardRead") -> ()  [unwired: 9 in, 1 out]
  n170 = call-poly <vilib>:"NT Write Value.vi"("Numeric"=w25, "Name"="ClimberEncoderDashBoardRead") -> ()  [unwired: 9 in, 1 out]
  n171 = call-poly <vilib>:"NT Write Value.vi"("Numeric"=w27, "Name"="ElevatorPositionDashBoardRead") -> ()  [unwired: 9 in, 1 out]
  n172 = call-poly <vilib>:"NT Write Value.vi"("Numeric"=w19, "Name"="ClimberStateDashBoardRead") -> ()  [unwired: 9 in, 1 out]
  n173 = global read "Robot Global Data.vi" "Hatch In?"() -> (w29:bool)
  n174 = global read "Robot Global Data.vi" "Cargo In?"() -> (w32:bool)
  n175 = global read "Robot Global Data.vi" "TracaoEsq"() -> (w18:dbl)
  n176 = global read "Robot Global Data.vi" "TracaoDir"() -> (w16:dbl)
  n177 = call <vilib>:"WPI_MotorControlRefNum Registry Get.vi"("refnum name"="Elevador1") -> ("MotorControlDevRef"=w54:T7)  [unwired: 9 in, 1 out]
  n178 = call <vilib>:"WPI_EncoderRefNum Registry Get.vi"("refnum name"="Elevador Encoder") -> ("error out"=w57:errorcluster, "EncoderDevRef"=w58:T17)  [unwired: 9 in]
  n179 = call <vilib>:"WPI_MotorControlRefNum Registry Get.vi"("refnum name"="Elevador2") -> ("MotorControlDevRef"=w53:T7)  [unwired: 9 in, 1 out]
  n180 = call-poly <vilib>:"NT Write Value.vi"("Boolean"=w29, "Name"="HatchDashBoardRead") -> ()  [unwired: 9 in, 1 out]
  n181 = disable-structure shown="Enabled" {
    disable-tunnel: w58 -> [w387 w414]
    disable-tunnel: w57 -> [w386 w413]
    disable-tunnel: w54 -> [_ w412]
    disable-tunnel: w53 -> [_ w411]
    frame Disabled {
      n182 = call <vilib>:"WPI_MotorControlRefNum Registry Get.vi"("refnum name"="Elevador1") -> ("error out"=w392:errorcluster, "MotorControlDevRef"=w393:T7)  [unwired: 9 in]
      n183 = call <vilib>:"WPI_MotorControlRefNum Registry Get.vi"("refnum name"="Elevador2") -> ("error out"=w388:errorcluster, "MotorControlDevRef"=w389:T7)  [unwired: 9 in]
      n184 = while {
        tunnel: w393 -> [w407]
        tunnel: w392 -> [w406]
        tunnel: w389 -> [w399]
        tunnel: w388 -> [w398]
        tunnel: w387 -> [w395]
        tunnel: w386 -> [w394]
        stop <- FALSE stop-if-true
        n185 = call <vilib>:"WPI_EncoderGet.vi"("error in (no error)"=w394, "EncoderDevRef"=w395) -> ()  [unwired: 4 in, 6 out]
        n186 = global read "Robot Global Data.vi" "D-Pad"() -> (w408:T24)
        n187 = Wait (ms)(milliseconds to wait=u32 50) -> ()  [unwired: 1 out]
        n188 = Unbundle By Name(w408) -> ("Top"=w405:bool, "Bottom"=w403:bool)
        n189 = Negate(x="Sobe") -> (-x=w400:dbl)
        n190 = Select(t=w400, s=w403, f=0.0) -> (s? t:f=w404:dbl)
        n191 = Select(t="Desce", s=w405, f=w404) -> (s? t:f=w397:dbl)
        n192 = call <vilib>:"WPI_MotorControlSetOutput.vi"("error in (no error)"=w406, "Output"=w397, "MotorControlDevRef"=w407) -> ()  [unwired: 6 in, 3 out]
        n193 = call <vilib>:"WPI_MotorControlSetOutput.vi"("error in (no error)"=w398, "Output"=w397, "MotorControlDevRef"=w399) -> ()  [unwired: 6 in, 3 out]
      }
    }
    frame Enabled {
      n194 = while {
        tunnel: w414 -> [w417]
        tunnel: w413 -> [w416]
        tunnel: w412 -> [w434]
        tunnel: w411 -> [w433]
        stop <- FALSE stop-if-true
        n195 = global read "Robot Global Data.vi" "Elevador Limit"() -> (w418:bool)
        n196 = call <vilib>:"WPI_EncoderGet.vi"("error in (no error)"=w416, "EncoderDevRef"=w417) -> ("Distance"=w415:dbl)  [unwired: 4 in, 5 out]
        "elavador  pos" <- w415
        n197 = global read "Robot Global Data.vi" "Setpoint Elevador"() -> (w427:dbl)
        n198 = global write "Robot Global Data.vi" "Elevador Height"(w415) -> ()
        n199 = case shown="True" w418 {
          tunnel: w417 -> [_ w437]
          tunnel: w416 -> [_ w436]
          frame False {
          }
          frame True {
            n200 = call <vilib>:"WPI_EncoderReset.vi"("error in (no error)"=w436, "EncoderDevRef"=w437) -> ()  [unwired: 8 in, 2 out]
          }
        }
        n201 = call "In Range.vi"("Range"=2.0, "Setpoint"=0.0, "Value"=w415) -> ("in range?"=w423:bool)  [unwired: 8 in]
        n202 = Equal To 0?(x=w427) -> (x = 0?=w426:bool)
        n203 = call "FancyPID.vi"("Gains"="Gains", "Range"="Range", "Disable Range"="Disable Range", "Integral Range"="Integral Range", "Process variable"=w415, "Setpoint"=w427) -> ("output"=w420:dbl)  [unwired: 5 in]
        n204 = And(x=w426, y=w423) -> (x .and. y?=w422:bool)
        n205 = Select(t=0.0, s=w422, f=w420) -> (s? t:f=w419:dbl)
        n206 = call <vilib>:"WPI_MotorControlSetOutput.vi"("Output"=w419, "MotorControlDevRef"=w434) -> ()  [unwired: 7 in, 3 out]
        n207 = call <vilib>:"WPI_MotorControlSetOutput.vi"("Output"=w419, "MotorControlDevRef"=w433) -> ()  [unwired: 7 in, 3 out]
        n208 = Wait (ms)(milliseconds to wait=u32 10) -> ()  [unwired: 1 out]
      }
    }
  }
  n209 = call-poly <vilib>:"NT Write Value.vi"("Boolean"=w32, "Name"="CargoDashBoardRead") -> ()  [unwired: 9 in, 1 out]
  n210 = call-poly <vilib>:"NT Write Value.vi"("Numeric"=w16, "Name"="TracaoDirDashBoardRead") -> ()  [unwired: 9 in, 1 out]
  n211 = call-poly <vilib>:"NT Write Value.vi"("Numeric"=w18, "Name"="TracaoEsqDashBoardRead") -> ()  [unwired: 9 in, 1 out]
  n212 = while {
    shift-right: [w452] -> _
    shift-left: Climber."Wait for Start" -> [w454]
    shift-right: [w448] -> _
    shift-left: 0.0 -> [w449]
    stop <- FALSE stop-if-true
    n213 = call <vilib>:"WPI_CompressorRefNum Registry Get.vi"("refnum name"="Compressor") -> ("error out"=w439:errorcluster, "CompressorDevRef"=w440:T25)  [unwired: 9 in]
    n214 = case shown="\"Charge\"" w454 {
      selector: w454 -> [w460 w473 w485 w496 w503 w510 w523 w532 _]
      tunnel: [w461 w474 w486 w497 w504 w511 w524 w533 Climber."cabou"] -> w452
      tunnel: [w457 _ w492 w498 w505 _ w518 "Retract back Speed" _] -> w451
      tunnel: [w457 _ w490 w498 w505 "Retract Speed" _ _ _] -> w450
      tunnel: w449 -> [_ w479 _ _ _ _ _ w530 _]
      tunnel: [_ w478 _ _ _ _ _ w529 _] -> w448
      tunnel: [_ 0.6 _ _ _ _ w525 _ _] -> w447
      tunnel: [_ 0.6 _ _ _ _ w525 _ _] -> w446
      tunnel: [_ _ _ _ TRUE TRUE TRUE TRUE TRUE] -> w442
      tunnel: [FALSE TRUE _ _ TRUE _ _ _ _] -> w441
      tunnel: w440 -> [_ w466 _ _ _ _ _ _ _]
      tunnel: w439 -> [_ w465 _ _ _ _ _ _ _]
      frame "Wait for Start", Default {
        w457 = 0.0
        n215 = global read "Robot Global Data.vi" "Buttons - Joy 0"() -> (w464:T12)
        n216 = Unbundle By Name(w464) -> ("Buttons[6]"=w463:bool, "Buttons[7]"=w462:bool)
        n217 = And(x=w463, y=w462) -> (x .and. y?=w458:bool)
        n218 = Select(t=Climber."Engaging Climb", s=w458, f=w460) -> (s? t:f=w461:T2)
      }
      frame "Engaging Climb" {
        n219 = call <vilib>:"WPI_CompressorStop.vi"("error in (no error)"=w465, "CompressorDevRef"=w466) -> ()  [unwired: 8 in, 2 out]
        n220 = global read "Robot Global Data.vi" "Buttons - Joy 0"() -> (w471:T12)
        n221 = Unbundle By Name(w471) -> ("Buttons[0]"=w468:bool)
        n222 = Increment(x=w479) -> (x+1=w478:dbl)
        n223 = Greater?(x=w478, y=2.0) -> (0:w469:bool)
        n224 = And(x=w468, y=w469) -> (x .and. y?=w470:bool)
        n225 = Select(t=Climber."ELEVATE!", s=w470, f=w473) -> (s? t:f=w474:T2)
      }
      frame "ELEVATE!" {
        n226 = global read "Robot Global Data.vi" "Climber Encoder"() -> (w488:dbl)
        n227 = global read "Robot Global Data.vi" "Climber Limit"() -> (w483:bool)
        n228 = Greater?(x=w488, y="Front Limit") -> (0:w484:bool)
        n229 = And(x=w484, y=w483) -> (x .and. y?=w482:bool)
        n230 = Select(t="Break speed", s=w484, f="Front Speed") -> (s? t:f=w490:dbl)
        n231 = Select(t="Break speed", s=w483, f="Back Speed") -> (s? t:f=w492:dbl)
        n232 = Select(t=Climber."Hold position", s=w482, f=w485) -> (s? t:f=w486:T2)
      }
      frame "Hold position" {
        n233 = global read "Robot Global Data.vi" "Buttons - Joy 0"() -> (w495:T12)
        n234 = Unbundle By Name(w495) -> ("Buttons[2]"=w494:bool)
        n235 = Select(t=Climber."Forward", s=w494, f=w496) -> (s? t:f=w497:T2)
        n236 = local read "Break speed"() -> (w498:dbl)
      }
      frame "Forward" {
        n237 = global read "Robot Global Data.vi" "Buttons - Joy 0"() -> (w500:T12)
        n238 = Unbundle By Name(w500) -> ("Buttons[3]"=w499:bool)
        n239 = Select(t=Climber."Retract varetas", s=w499, f=w503) -> (s? t:f=w504:T2)
        n240 = local read "Break speed"() -> (w505:dbl)
      }
      frame "Retract varetas" {
        n241 = global read "Robot Global Data.vi" "Climber Encoder"() -> (w513:dbl)
        n242 = Greater?(x=w513, y="Retract Distance") -> (0:w509:bool)
        n243 = Select(t=Climber."Charge", s=w509, f=w510) -> (s? t:f=w511:T2)
      }
      frame "Charge" {
        w525 = 0.4
        n244 = global read "Robot Global Data.vi" "Buttons - Joy 0"() -> (w521:T12)
        n245 = Unbundle By Name(w521) -> ("Buttons[1]"=w520:bool, "Buttons[2]"=w515:bool)
        n246 = Select(t=Climber."Sobe so um poquinho", s=w520, f=w523) -> (s? t:f=w524:T2)
        n247 = Select(t=0.9, s=w515, f=0.0) -> (s? t:f=w518:dbl)
      }
      frame "Sobe so um poquinho" {
        n248 = Increment(x=w530) -> (x+1=w529:dbl)
        n249 = Greater?(x=w529, y=10.0) -> (0:w531:bool)
        n250 = Select(t=Climber."cabou", s=w531, f=w532) -> (s? t:f=w533:T2)
      }
      frame "cabou" {
        # "É nois valeu falou"
      }
    }
    n251 = call <vilib>:"WPI_JoystickRefNum Registry Get.vi"("refnum name"="Joystick 0") -> ("error out"=w444:errorcluster, "JoystickDevRef"=w445:T26)  [unwired: 9 in]
    n252 = global write "Robot Global Data.vi" "Back Speed"(w451) -> ()
    n253 = global write "Robot Global Data.vi" "Front Speed"(w450) -> ()
    n254 = Wait (ms)(milliseconds to wait=u32 100) -> ()  [unwired: 1 out]
    n255 = global write "Robot Global Data.vi" "Climber Pivot"(w442) -> ()
    n256 = global write "Robot Global Data.vi" "Reset Climber Encoder"(w441) -> ()
    n257 = call <vilib>:"WPI_JoystickSetOutputs.vi"("error in (no error)"=w444, "Right Rumble"=w446, "Left Rumble"=w447, "JoystickDevRef"=w445) -> ()  [unwired: 6 in, 2 out]
    "Climber State" <- w454
  }
  n258 = call <vilib>:"Get_Continuous_Angle.vi"("Device Number"=FRIC_navX_DeviceNumbersTypeDef."Dev0") -> ("Continuous Angle"=w14:T28)  [unwired: 10 in]
  n259 = Unbundle(w14) -> ("Rollover"=w12:dbl, "Yaw"=w11:dbl, "Cont Yaw"=w10:dbl)
  n260 = call-poly <vilib>:"NT Write Value.vi"("Numeric"=w10, "Name"="ContYawDashBoardRead") -> ()  [unwired: 9 in, 1 out]
  n261 = call-poly <vilib>:"NT Write Value.vi"("Numeric"=w12, "Name"="RolloverDashBoardRead") -> ()  [unwired: 9 in, 1 out]
  n262 = call-poly <vilib>:"NT Write Value.vi"("Numeric"=w11, "Name"="YawDashBoardRead") -> ()  [unwired: 9 in, 1 out]
